vi "Read SH-Persis (No Objects).vi"(8 "error in (no error)":errorcluster, 11 "Cluster In":T4={"Field"=0.0, "Rate"=0.0, "Status"={"Sweeping"=FALSE, "Clamped"=FALSE, "Hold"=FALSE, "At Rest"=FALSE, "Quench"=FALSE, "Persistent Mode"=FALSE, "Switch Heater"=FALSE}, "ILM Shut Down?"=FALSE, "IO Info"={"Address"={"Com Port"=1, "ISOBUS Address"=2, "GPIB Address"=24, "Communication"=enum."ISOBUS"}, "Version"=enum."IPS"}, "IO Info (Level Meter)"={"Address"={"Com Port"=1, "ISOBUS Address"=5, "GPIB Address"=24, "Communication"=enum."ISOBUS"}, "ILM Name"="", "Display Channel"=[]}, "Training?"=FALSE, "Training Field and Speed Cluster"={"Training Field"=[0.0, 4.108, 5.78, 8.001], "Training Speed"=[0.0057, 0.0022833333333333334, 0.0011333333333333334, 0.0011333333333333334]}}) -> (0 "error out":errorcluster, 1 "SHon?":bool, 2 "pers?":bool, 3 "Cluster Out":T4={"Field"=0.0, "Rate"=0.0, "Status"={"Sweeping"=FALSE, "Clamped"=FALSE, "Hold"=FALSE, "At Rest"=FALSE, "Quench"=FALSE, "Persistent Mode"=FALSE, "Switch Heater"=FALSE}, "ILM Shut Down?"=FALSE, "IO Info"={"Address"={"Com Port"=1, "ISOBUS Address"=2, "GPIB Address"=24, "Communication"=enum."ISOBUS"}, "Version"=enum."IPS"}, "IO Info (Level Meter)"={"Address"={"Com Port"=1, "ISOBUS Address"=5, "GPIB Address"=24, "Communication"=enum."ISOBUS"}, "ILM Name"="", "Display Channel"=[]}, "Training?"=FALSE, "Training Field and Speed Cluster"={"Training Field"=[0.0, 4.108, 5.78, 8.001], "Training Speed"=[0.0057, 0.0022833333333333334, 0.0011333333333333334, 0.0011333333333333334]}}, 4 "Switch Heater":T6={"Value"=1, "Off (at zero field)"=FALSE, "On"=TRUE, "Off (at field)"=FALSE, "No switch fitted"=FALSE, "Confirm"=FALSE}, 5 "SHstatus":T5)   [LabVIEW 2012]
uses:
  Switch Heater Status.ctl
  Magnet status.ctl
  Oxford/PSSUBS.LLB/PSIO.ctl
  Oxford/BUSGEN.LLB/OxfordAddress.ctl
  Power Supply.lvclass
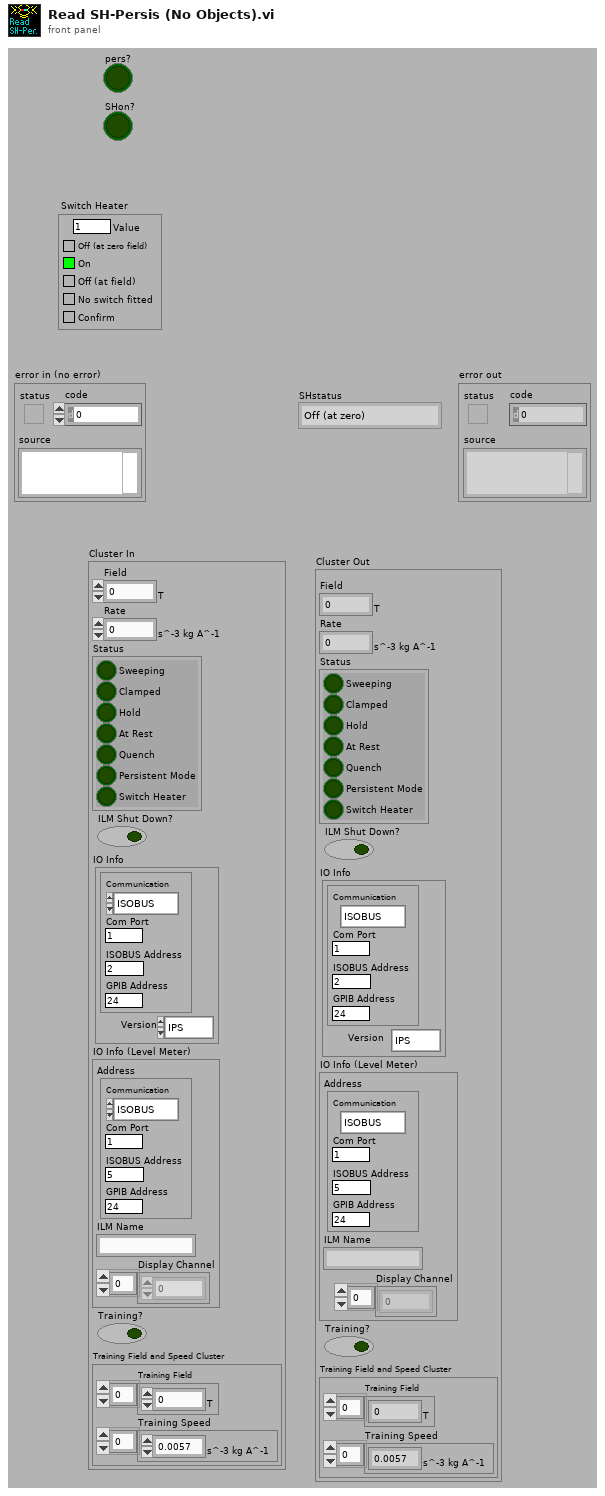
[diagram p1: front panel]
types:
  T1 = typedef "Power Supply.lvclass/Magnet status.ctl" = cluster{"Sweeping":bool, "Clamped":bool, "Hold":bool, "At Rest":bool, "Quench":bool, "Persistent Mode":bool, "Switch Heater":bool}
  T2 = typedef "PSIO.ctl" = cluster{"Address":T3, "Version":enum16{"PS", "IPS"}}
  T3 = typedef "OxfordAddress.ctl" = cluster{"Com Port":i32, "ISOBUS Address":i32, "GPIB Address":i16, "Communication":enum16{"RS232", "ISOBUS", "GPIB", "Gateway"}}
  T4 = cluster{"Field":dbl[unit], "Rate":dbl[unit], "Status":T1, "ILM Shut Down?":bool, "IO Info":T2, "IO Info (Level Meter)":cluster{"Address":T3, "ILM Name":string, "Display Channel":i32[]}, "Training?":bool, "Training Field and Speed Cluster":cluster{"Training Field":dbl[unit][], "Training Speed":dbl[unit][]}}
  T5 = typedef "Power Supply.lvclass/Switch Heater Status.ctl" = enum16{"Off (at zero)", "On", "Off (at field)", "Other"}
  T6 = cluster{"Value":i16, "Off (at zero field)":bool, "On":bool, "Off (at field)":bool, "No switch fitted":bool, "Confirm":bool}
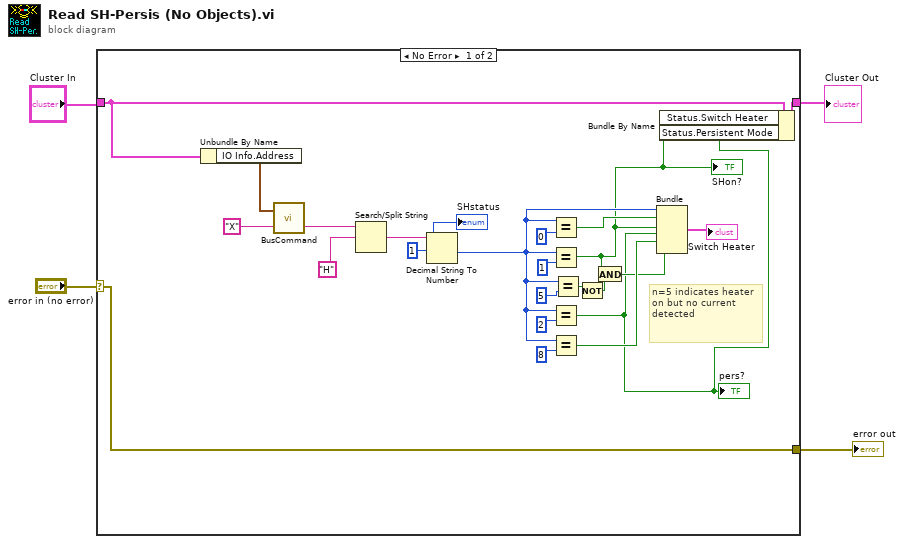
[diagram p0: block diagram]
diagram:
  n1 = case shown="No Error" "error in (no error)" {
    selector: "error in (no error)" -> [w9 w28]
    tunnel: "Cluster In" -> [w10 w29]
    tunnel: [w8 w29] -> w1
    tunnel: [w9 w28] -> w3
    frame No Error {
      # "n=5 indicates heater on but no current detected"
      n2 = Unbundle By Name(w10) -> ("IO Info.Address"=w14:T3)
      n3 = call "BusCommand.vi"("Command"="X", "Instrument address (in)"=w14) -> ("Reply"=w19:string)  [unwired: 1 out]
      n4 = Search/Split String(string=w19, search string/char (-)="H") -> (match + rest of string=w26:string)  [unwired: 3 out]
      n5 = Decimal String To Number(string=w26, offset=1) -> (number=w11:i32)  [unwired: 2 out]
      "SHstatus" <- w11
      n6 = Equal?(x=w11, y=0) -> (x = y?=w23:bool)
      n7 = Equal?(x=w11, y=1) -> (x = y?=w6:bool)
      "SHon?" <- w6
      n8 = Equal?(x=w11, y=2) -> (x = y?=w5:bool)
      "pers?" <- w5
      n9 = Equal?(x=w11, y=8) -> (x = y?=w20:bool)
      n10 = Equal?(x=w11, y=5) -> (x = y?=w15:bool)
      n11 = Not(x=w15) -> (.not. x?=w16:bool)
      n12 = And(x=w6, y=w16) -> (x .and. y?=w18:bool)
      n13 = Bundle(w11, w23, w6, w5, w20, w18) -> (→"Switch Heater":cluster{i32, bool, bool, bool, bool, bool})  [unwired: 1 out]
      n14 = Bundle By Name(cluster=w10, "Status.Switch Heater"=w6, "Status.Persistent Mode"=w5) -> (w8:T4)
    }
    frame Error {
    }
  }
  "error out" <- w3
  "Cluster Out" <- w1
